vi "test_Write Digital WSS Out.vi"(8 "error in (no error)":errorcluster, 11 "TestCase in":refnum<class "FPGA Addon Speciality IO Tests.lvclass">) -> (0 "error out":errorcluster, 3 "TestCase out":refnum<class "FPGA Addon Speciality IO Tests.lvclass">)   [LabVIEW 2021, in "FPGA Addon Speciality IO Tests.lvclass"]
uses:
  FPGA Addon Speciality IO Tests.lvclass
  C:/Program Files/National Instruments/LabVIEW 2021/vi.lib/NI/VeriStand Custom Device Testing Tools/VeriStandTestCase/VeriStandTestCase.lvclass
  <vilib>/addons/_JKI Toolkits/VI Tester/TestCase.llb/TestCase.lvclass
  FPGA Addon Test Class/FPGA Addon Test Class.lvclass
  C:/Program Files/National Instruments/LabVIEW 2021/vi.lib/addons/_JKI Toolkits/VI Tester/TestCase.llb/TestCase.lvclass
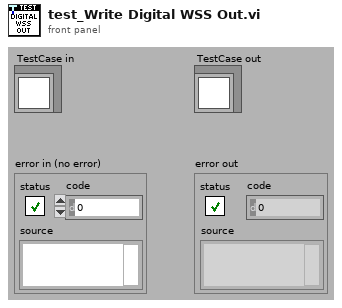
[diagram p1: front panel]
types:
  T1 = typedef "NI_VS Workspace ExecutionAPI.lvlib/WorkspaceAPI.ctl" = refnum<k24>
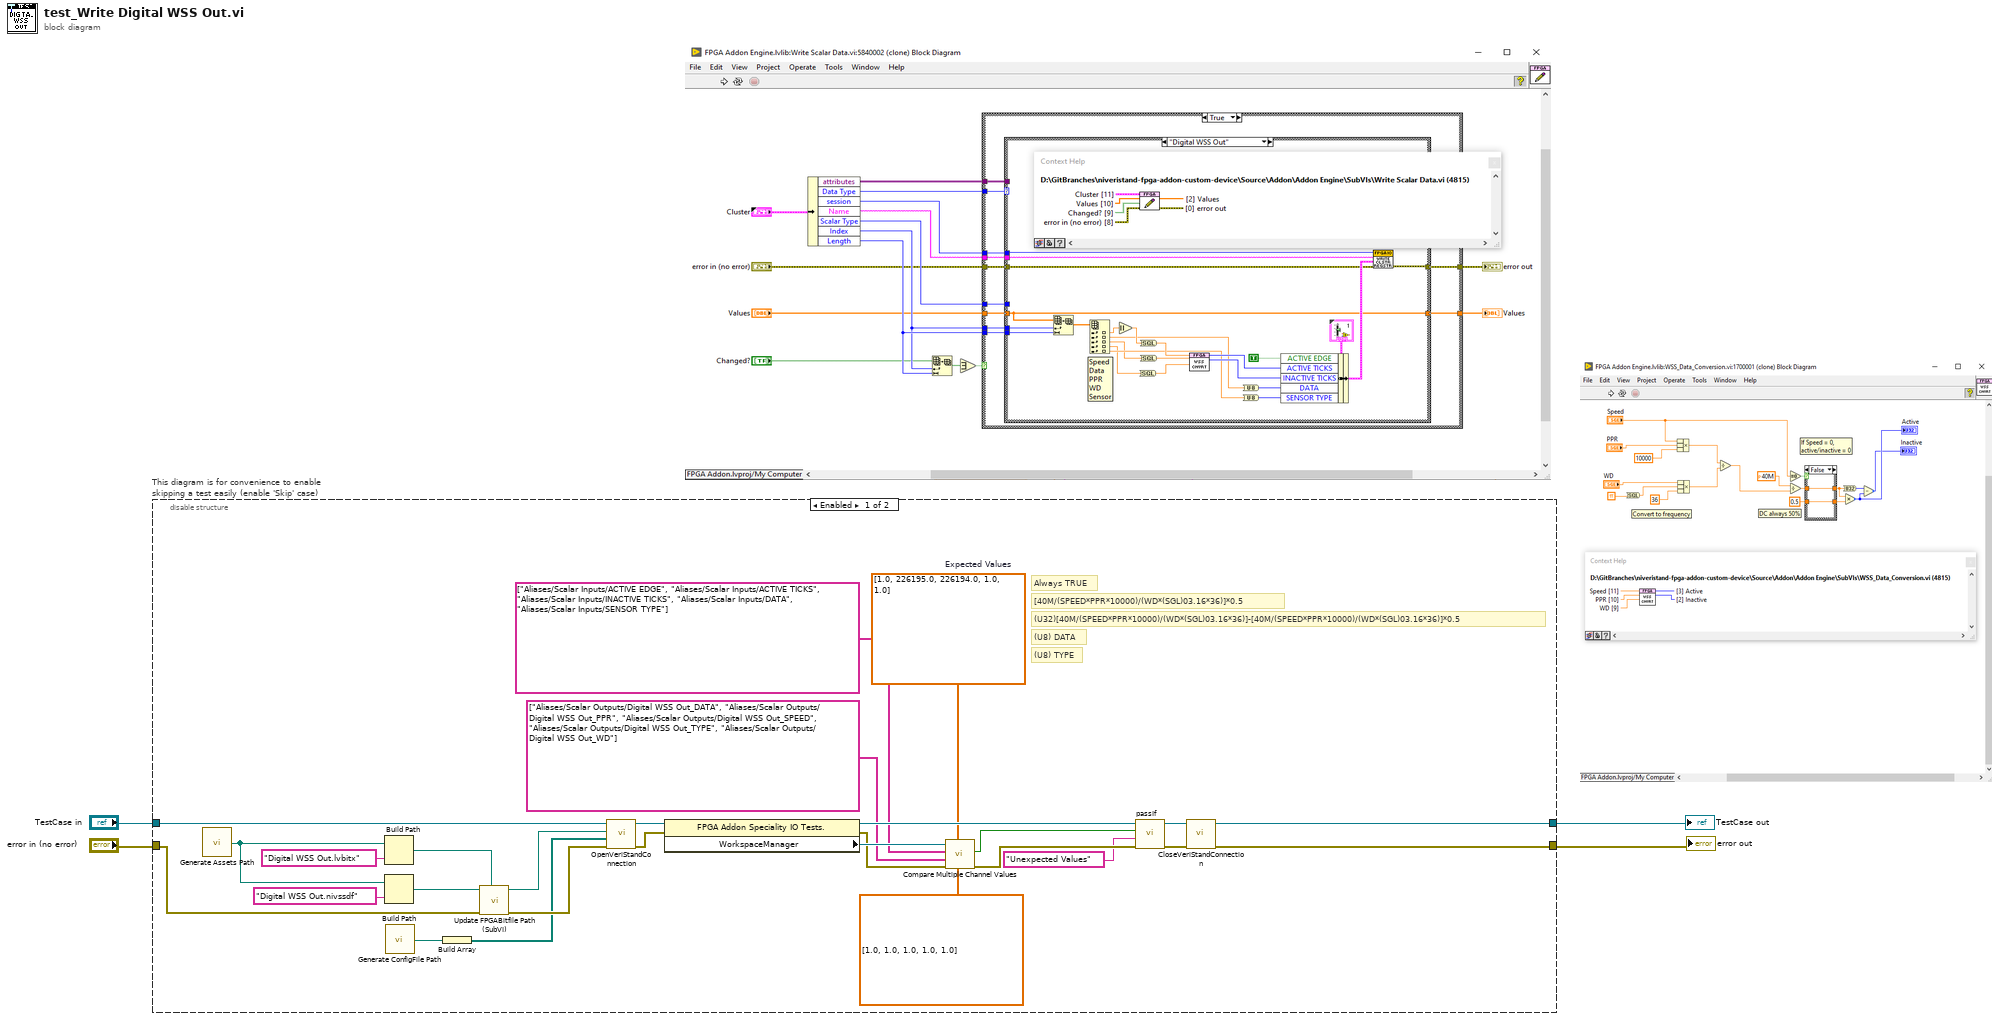
[diagram p0: block diagram]
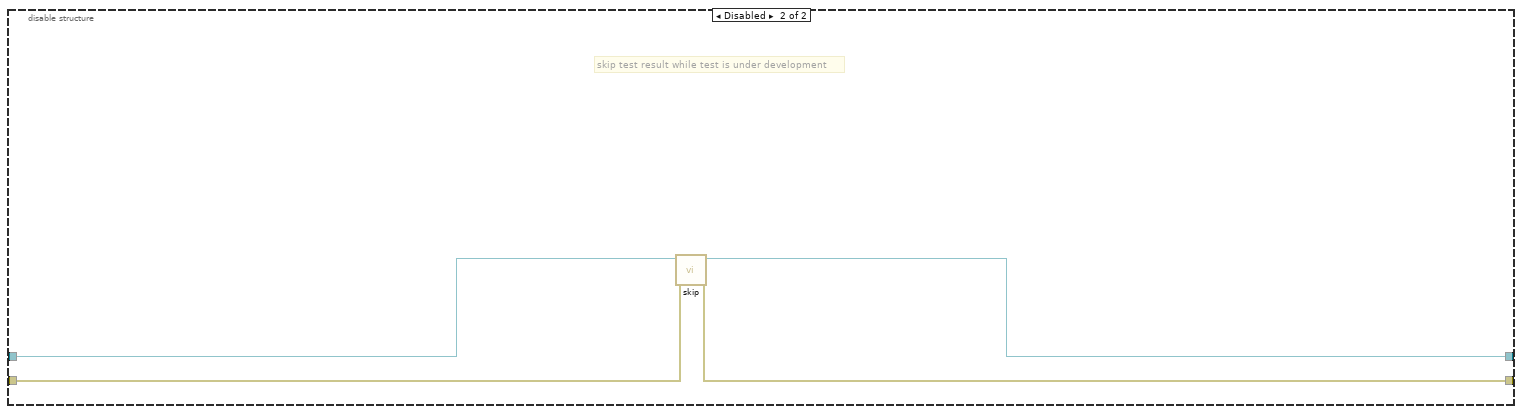
[diagram p2: hidden frame]
diagram:
  n1 = disable-structure "This diagram is for convenience to enable skipping a test easily (enable 'Skip' case)" shown="Enabled" {
    disable-tunnel: "TestCase in" -> [w29 w35]
    disable-tunnel: [w27 w33] -> w1
    disable-tunnel: [w28 w34] -> w3
    disable-tunnel: "error in (no error)" -> [w10 w32]
    frame Enabled {
      w18 = dbl[] [1.0, 226195.0, 226194.0, 1.0, 1.0]  # Expected Values
      # "(U32)[40M/(SPEED*PPR*10000)/(WD*(SGL)03.16*36)]-[40M/(SPEED*PPR*10000)/(WD*(SGL)03.16*36)]*0.5"
      # "[40M/(SPEED*PPR*10000)/(WD*(SGL)03.16*36)]*0.5"
      # "(U8) TYPE"
      # "(U8) DATA"
      # "Always TRUE"
      n2 = call "Generate Assets Path.vi"() -> ("Assets path"=w13:path)
      n3 = Build Path(base path=w13, name or relative path="Digital WSS Out.lvbitx") -> (appended path=w12:path)
      n4 = Build Path(base path=w13, name or relative path="Digital WSS Out.nivssdf") -> (appended path=w11:path)
      n5 = call "Generate ConfigFile Path.vi"() -> ("ConfigFile path"=w14:path)
      n6 = Build Array(w14) -> (w7:path[])
      n7 = call "Update FPGABitfile Path (SubVI).vi"("Bitfile Path"=w12, "error in (no error)"=w10, "System Definition path in"=w11) -> ("error out"=w9:errorcluster, "System Definition path out"=w8:path)  [unwired: 7 in]
      n8 = call-dynamic "OpenVeriStandConnection.vi"("error in (no error)"=w9, "overrides files"=w7, "System Definition File"=w8, "VeriStand Test Case in"=w29) -> ("error out"=w31:errorcluster, "VeriStand Test Case out"=w30:refnum<class "FPGA Addon Speciality IO Tests.lvclass">)  [unwired: 5 in, 1 out]
      n9 = property class="FPGA Addon Speciality IO Tests."(reference=w30, error in=w31) -> (reference out=w26:refnum<class "FPGA Addon Speciality IO Tests.lvclass">, error out=w22:errorcluster, "WorkspaceManager"=w23:T1)
      n10 = call "Compare Multiple Channel Values.vi"("Values"=dbl[] [1.0, 1.0, 1.0, 1.0, 1.0], "Expected Values"=w18, "error in (no error)"=w22, "Scalar Outputs"=string[] ["Aliases/Scalar Outputs/Digital WSS Out_DATA", "Aliases/Scalar Outputs/Digital WSS Out_PPR", "Aliases/Scalar Outputs/Digital WSS Out_SPEED", "Aliases/Scalar Outputs/Digital WSS Out_TYPE", "Aliases/Scalar Outputs/Digital WSS Out_WD"] ("Channels"), "Scalar Inputs"=string[] ["Aliases/Scalar Inputs/ACTIVE EDGE", "Aliases/Scalar Inputs/ACTIVE TICKS", "Aliases/Scalar Inputs/INACTIVE TICKS", "Aliases/Scalar Inputs/DATA", "Aliases/Scalar Inputs/SENSOR TYPE"] ("Channels"), ".NET Refnum in"=w23) -> ("error out"=w17:errorcluster, "Equals?"=w16:bool)  [unwired: 4 in]
      n11 = call-dynamic "passIf.vi"("error in (no error)"=w17, "message (\"\")"="Unexpected Values" ("message (\"\")"), "pass"=w16, "TestCase in"=w26) -> ("error out"=w24:errorcluster, "TestCase out"=w25:refnum<class "FPGA Addon Speciality IO Tests.lvclass">)  [unwired: 6 in]
      n12 = call-dynamic "CloseVeriStandConnection.vi"("error in (no error)"=w24, "VeriStand Test Case in"=w25) -> ("error out"=w28:errorcluster, "VeriStand Test Case out"=w27:refnum<class "FPGA Addon Speciality IO Tests.lvclass">)  [unwired: 8 in]
    }
    frame Disabled {
      # "skip test result while test is under development"
      n13 = call <vilib>:"skip.vi"("error in (no error)"=w32, "TestCase in"=w35) -> ("error out"=w34:errorcluster, "TestCase out"=w33:refnum<class "FPGA Addon Speciality IO Tests.lvclass">)  [unwired: 8 in]
    }
  }
  "error out" <- w3
  "TestCase out" <- w1
